vi "SPI_SetThreeWire.vi"(5 "Device":i32, 6 "Three Wire":bool, 7 "Bus":i32=1, 8 "error in":errorcluster) -> (0 "error out":errorcluster)   [LabVIEW 2014]
doc: "Select whether or not to share the SI/SO lines for the specified SPI device. Default is to use separate lines."
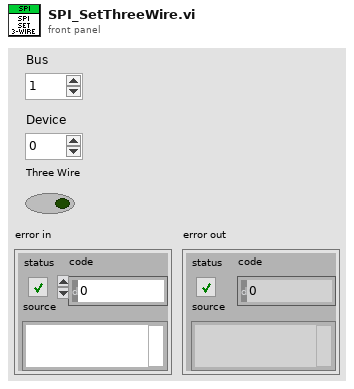
[diagram p1: front panel]
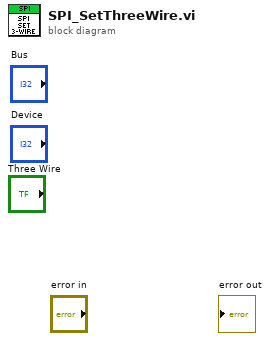
[diagram p0: block diagram]
diagram:
